vi "GetDescription.vi"(8 "error in (no error)":errorcluster caption="错误输入（无错误）", 11 "CondimentDecorator 输入":refnum<class "CondimentDecorator.lvclass">) -> (0 "error out":errorcluster caption="错误输出", 2 "Description":string, 3 "CondimentDecorator 输出":refnum<class "CondimentDecorator.lvclass">)   [LabVIEW 2016, in "CondimentDecorator.lvclass"]
uses:
  CondimentDecorator.lvclass
  Beverage.lvclass
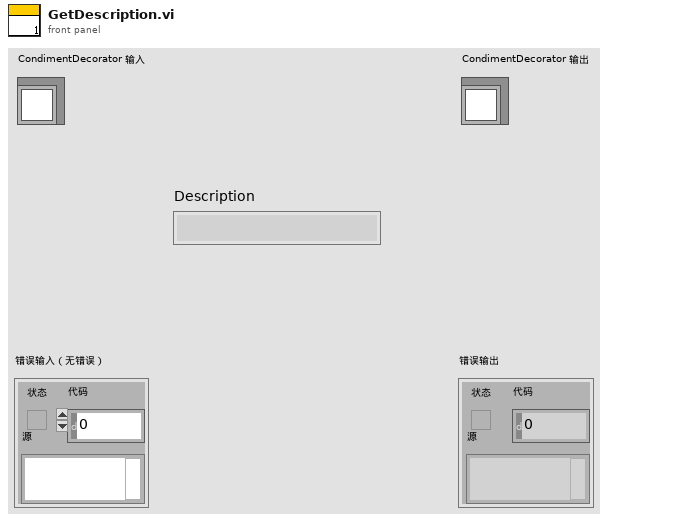
[diagram p1: front panel]
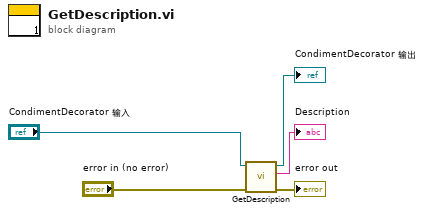
[diagram p0: block diagram]
diagram:
  n1 = call-parent "GetDescription.vi"("error in (no error)"="error in (no error)", "Beverage 输入"="CondimentDecorator 输入") -> ("error out"=→"error out":errorcluster, "Description"=→"Description":string, "Beverage 输出"=→"CondimentDecorator 输出":refnum<class "CondimentDecorator.lvclass">)  [unwired: 7 in]
